vi "UnInit Globals.vi"(8 "error in":errorcluster) -> (0 "error out":errorcluster)   [LabVIEW 2020, in "Netatmo-WeatherStation.lvlib"]
uses:
  Netatmo-WeatherStation.lvlib
  globals.vi
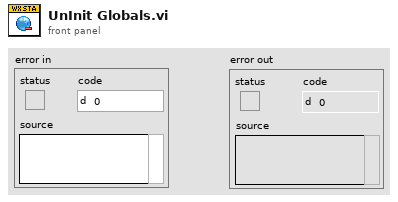
[diagram p1: front panel]
types:
  T1 = cluster{"Redirect Data":refnum<user-event>, "Redirect Error":refnum<user-event>}
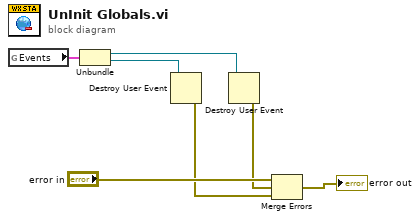
[diagram p0: block diagram]
diagram:
  n1 = global read "globals.vi" "Events"() -> (w6:T1)
  n2 = Unbundle(w6) -> ("Redirect Data"=w4:refnum<user-event>, "Redirect Error"=w5:refnum<user-event>)
  n3 = Destroy User Event(user event=w5) -> (error out=w1:errorcluster)  [unwired: 1 in]
  n4 = Destroy User Event(user event=w4) -> (error out=w2:errorcluster)  [unwired: 1 in]
  n5 = Merge Errors("error in", w2, w1) -> (→"error out":errorcluster)
